vi "Handle Messages.vi"(8 "error in (no error)":errorcluster, 9 "Message Data":variant, 10 "Message":string, 11 "Barista In":refnum<class "Barista.lvclass">) -> (0 "error out":errorcluster, 3 "Barista Out":refnum<class "Barista.lvclass">)   [LabVIEW 2020, in "Barista.lvclass"]
uses:
  Barista.lvclass
  C:/Users/anton/Documents/GitHub/Triarc-Examples/Coffee Shop/Person/Person.lvclass
  Support/Order Item/Order Item.lvclass
  Worker/Worker.lvclass
  Person/Person.lvclass
  C:/Users/anton/Documents/GitHub/Triarc-Examples/Coffee Shop/Worker/Worker.lvclass
  C:/Program Files (x86)/National Instruments/LabVIEW 2020/vi.lib/Asteme/Triarc Framework/View/View.lvclass
  C:/Program Files (x86)/National Instruments/LabVIEW 2020/vi.lib/Asteme/Triarc Framework/Process/Process.lvclass
  C:/Program Files (x86)/National Instruments/LabVIEW 2020/vi.lib/Asteme/Triarc Framework/Base/Base.lvclass
  C:/Program Files (x86)/National Instruments/LabVIEW 2020/vi.lib/Asteme/Triarc Framework/Error Handler Interface/Error Handler Interface.lvclass
  C:/Program Files (x86)/National Instruments/LabVIEW 2020/vi.lib/Asteme/Triarc Framework/Logging/Logging.lvclass
  C:/Users/anton/Documents/GitHub/Triarc-Examples/Coffee Shop/Process Job/Job Handler.lvclass
  C:/Users/anton/Documents/GitHub/Triarc-Examples/Coffee Shop/Barista/Barista.lvclass
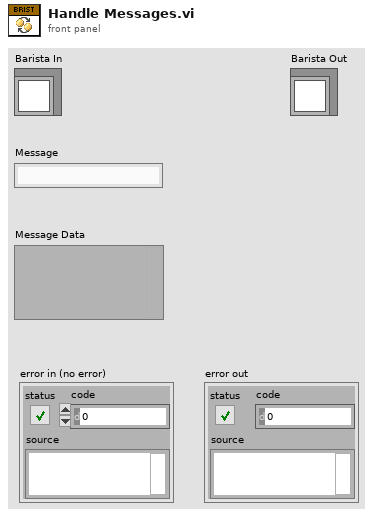
[diagram p1: front panel]
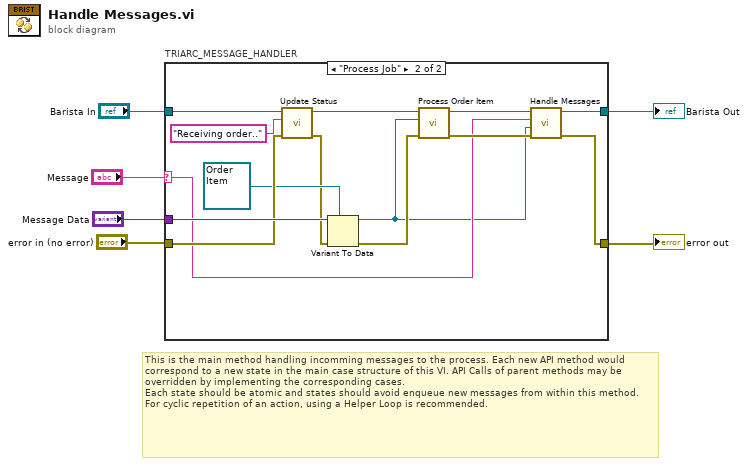
[diagram p0: block diagram]
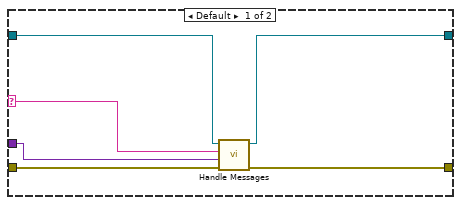
[diagram p2: hidden frame]
diagram:
  # "This is the main method handling incomming messages to the process. Each new API method would correspond to a new state in the main case structure of this VI. API Calls of parent methods may be overridden by implementing the corresponding cases.\nEach state should be atomic and states should avoid enqueue new messages from within this method. For cyclic repetition of an action, using a Helper Loop is recommended."
  n1 = case "TRIARC_MESSAGE_HANDLER" shown="\"Process Job\"" "Message" {
    selector: "Message" -> [w10 w18]
    tunnel: "error in (no error)" -> [w9 w25]
    tunnel: "Barista In" -> [w12 w15]
    tunnel: "Message Data" -> [w11 w26]
    tunnel: [w8 w21] -> w2
    tunnel: [w7 w19] -> w1
    frame Default {
      n2 = call-parent "Handle Messages.vi"("error in (no error)"=w9, "Message Data"=w11, "Message"=w10, "Worker In"=w12) -> ("error out"=w8:errorcluster, "Worker Out"=w7:refnum<class "Barista.lvclass">)  [unwired: 6 in]
    }
    frame "Process Job" {
      n3 = call "Update Status.vi"("error in (no error)"=w25, "Status"="Receiving order..", "Person In"=w15) -> ("error out"=w16:errorcluster, "Person Out"=w14:refnum<class "Barista.lvclass">)  [unwired: 7 in]
      n4 = Variant To Data(error in=w16, type=refnum<class "Order Item.lvclass"> refnum ("Order Item.lvclass"), Variant=w26) -> (data=w17:refnum<class "Order Item.lvclass">, error out=w23:errorcluster)
      n5 = call "Process Order Item.vi"("error in (no error)"=w23, "Order Item.lvclass"=w17, "Barista in"=w14) -> ("error out"=w22:errorcluster, "Barista out"=w20:refnum<class "Barista.lvclass">)  [unwired: 7 in]
      n6 = call-parent "Handle Messages.vi"("error in (no error)"=w22, "Message Data"=w17, "Message"=w18, "Worker In"=w20) -> ("error out"=w21:errorcluster, "Worker Out"=w19:refnum<class "Barista.lvclass">)  [unwired: 6 in]
    }
  }
  "error out" <- w2
  "Barista Out" <- w1
